vi "setDataValueStep.vi"(8 "error in (no error)":errorcluster, 10 "dataValueStep":dbl, 11 "RampEvent.lvclass in":refnum<class "RampEvent.lvclass">) -> (0 "error out":errorcluster, 3 "RampEvent.lvclass out":refnum<class "RampEvent.lvclass">)   [LabVIEW 2011, in "Tools.lvlib" / "Scripting.lvlib" / "RampEvent.lvclass"]
uses:
  RampEvent.lvclass
  RampEvent.lvclass/RampEvent.ctl
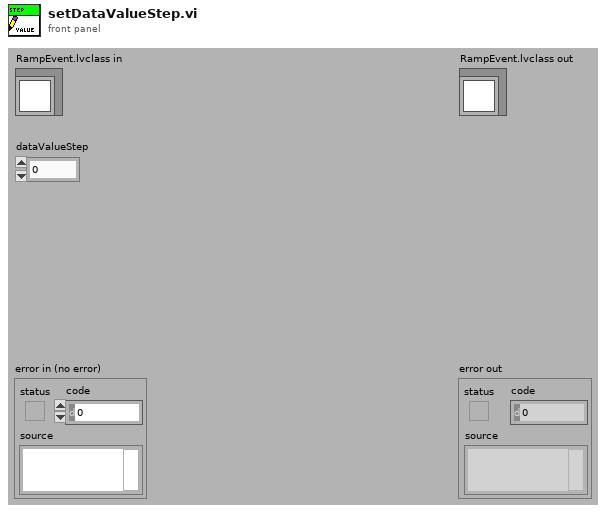
[diagram p1: front panel]
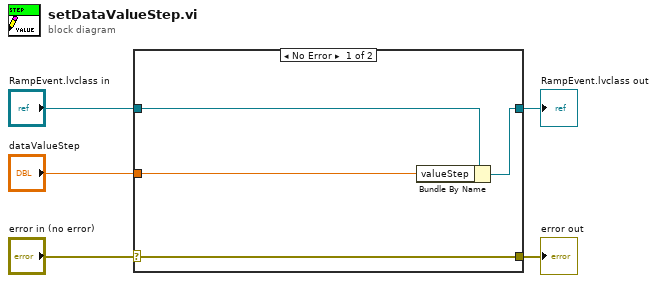
[diagram p0: block diagram]
diagram:
  n1 = case shown="No Error" "error in (no error)" {
    selector: "error in (no error)" -> [w9 w10]
    tunnel: [w9 w10] -> w4
    tunnel: [w7 w11] -> w2
    tunnel: "RampEvent.lvclass in" -> [w8 w11]
    tunnel: "dataValueStep" -> [w6 _]
    frame No Error {
      n2 = Bundle By Name(cluster=w8, "valueStep"=w6) -> (w7:refnum<class "RampEvent.lvclass">)
    }
    frame Error {
    }
  }
  "error out" <- w4
  "RampEvent.lvclass out" <- w2
